vi "UV-VIS SetExposureTime.vi"(3 "error in (no error)":errorcluster, 4 "time":sgl format="%.2f", 5 "Control in":refnum<class "CCD_camera.lvclass">) -> (0 "error out":errorcluster, 1 "DLL error code":u32, 2 "Control out":refnum<class "CCD_camera.lvclass">)   [LabVIEW 2020, in "CCD_camera.lvclass"]
doc: "This function will set the exposure time to the nearest valid value not less than the given value. The actual exposure time used is obtained by <B>GetAcquisitionTimings</B>. See section on Acquisition Modes for further details.\n\n<B>Parameter:</B>\ntime - the exposure time in seconds.\n\n<B>Error codes:</B>\nDRV_SUCCESS - Exposure time accepted.\nDRV_NOT_INITIALIZED - System not initialized.\nDRV_ACQUIRING - Acquisition in progress.\nDRV_P1INVALID - Exposure Time invalid.\n\n<B>NOTES:</B>\n<B>If the current acquisition mode is Single-track, Multi-Track or Image then this function will actually set the shutter time. The actual exposure time used is obtained from GetAcquisitionTimings.</B>"
uses:
  CCD_camera.lvclass
  C:/dev/TRANCON/Classes/Detector/Detector.lvclass
  Detector.lvclass/Detector.ctl
  Detector.lvclass
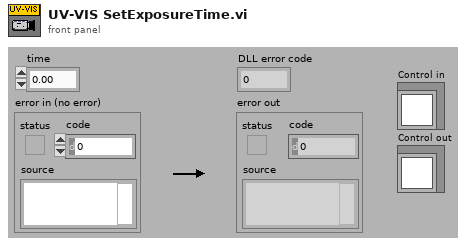
[diagram p1: front panel]
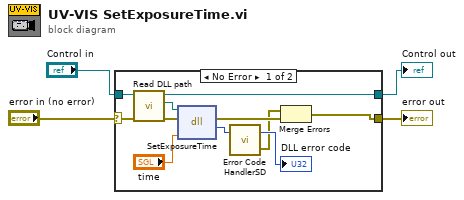
[diagram p0: block diagram]
diagram:
  n1 = case shown="No Error" "error in (no error)" {
    selector: "error in (no error)" -> [w6 w17]
    tunnel: [w8 w17] -> w3
    tunnel: [w5 w16] -> w2
    tunnel: "Control in" -> [w7 w16]
    frame No Error {
      n2 = call "Read DLL path.vi"("error in (no error)"=w6, "Detector in"=w7) -> ("error out"=w11:errorcluster, "DLL path"=w12:path, "Detector out"=w5:refnum<class "CCD_camera.lvclass">)  [unwired: 7 in]
      n3 = dll-call lib="S:/TRANCON/DLL/Atmcd32d.dll" fn="SetExposureTime"(path in=w12, error in=w11, "time"="time") -> (error out=w10:errorcluster, "return type"=w15:u32)  [unwired: 2 in, 1 out]
      n4 = call "Error Code HandlerSD.vi"("DLL error code"=w15) -> ("error out"=w9:errorcluster, "dup DLL error code"=→"DLL error code":u32)  [unwired: 1 in]
      n5 = Merge Errors(w9, w10) -> (w8:errorcluster)
    }
    frame Error {
    }
  }
  "error out" <- w3
  "Control out" <- w2
